vi "Motor_Calibrate.vi"() -> ()   [LabVIEW 2009, in "Motor.lvlib"]
uses:
  Motor.lvlib
  PWM/PWM_Name.ctl
  FPGA.lvlib
  PWM.lvlib
panel:
  in  "stop":bool
  in  "start":bool
  in  "PWM_Channel":T1=1 items=["Invalid"=0, "PWM1"=1, "PWM2"=2, "PWM9"=9, "PWM10"=10]
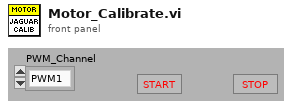
[diagram p1: front panel]
types:
  T1 = typedef "PWM.lvlib/PWM_Name.ctl" = u16
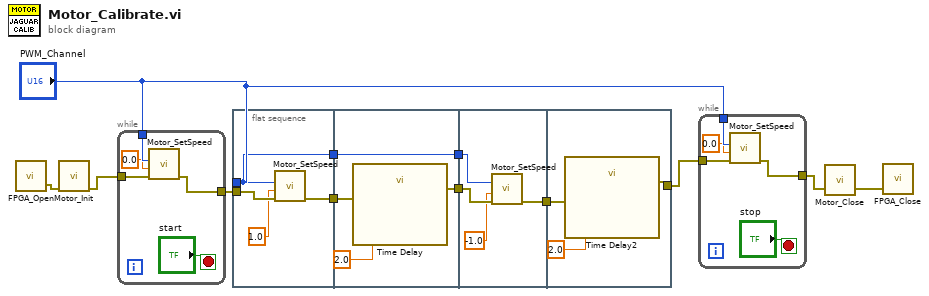
[diagram p0: block diagram]
diagram:
  n1 = call "FPGA_Open.vi"() -> ("error out"=w12:errorcluster)  [unwired: 3 in]
  n2 = call "Motor_Init.vi"("error in"=w12) -> ("error out"=w5:errorcluster)  [unwired: 10 in]
  n3 = while {
    tunnel: w5 -> [w16]
    tunnel: [w15] -> w4
    tunnel: "PWM_Channel" -> [w14]
    stop <- "start" stop-if-true
    n4 = call "Motor_SetSpeed.vi"("error in"=w16, "Speed"=0.0, "PWM_Channel"=w14) -> ("error out"=w15:errorcluster)  [unwired: 8 in]
  }
  n5 = flat-sequence {
    tunnel: w4 -> [w21]
    tunnel: "PWM_Channel" -> [w18]
    tunnel: [w19] -> w10
    tunnel: [w18] -> w7
    tunnel: w10 -> [w25]
    tunnel: [w24] -> w9
    tunnel: [w22] -> w8
    tunnel: w7 -> [w22]
    tunnel: w9 -> [w28]
    tunnel: w8 -> [w29]
    tunnel: [w26] -> w6
    tunnel: [w31] -> w3
    tunnel: w6 -> [w32]
    frame #0 {
      n6 = call "Motor_SetSpeed.vi"("error in"=w21, "Speed"=1.0, "PWM_Channel"=w18) -> ("error out"=w19:errorcluster)  [unwired: 8 in]
    }
    frame #1 {
      n7 = call "Time Delay"("error in (no error)"=w25, "Delay Time (s)"=2.0) -> ("error out"=w24:errorcluster)  [unwired: 9 in]
    }
    frame #2 {
      n8 = call "Motor_SetSpeed.vi"("error in"=w28, "Speed"=-1.0, "PWM_Channel"=w29) -> ("error out"=w26:errorcluster)  [unwired: 8 in]
    }
    frame #3 {
      n9 = call "Time Delay2"("error in (no error)"=w32, "Delay Time (s)"=2.0) -> ("error out"=w31:errorcluster)  [unwired: 9 in]
    }
  }
  n10 = while {
    tunnel: w3 -> [w36]
    tunnel: [w35] -> w2
    tunnel: "PWM_Channel" -> [w34]
    stop <- "stop" stop-if-true
    n11 = call "Motor_SetSpeed.vi"("error in"=w36, "Speed"=0.0, "PWM_Channel"=w34) -> ("error out"=w35:errorcluster)  [unwired: 8 in]
  }
  n12 = call "Motor_Close.vi"("error in"=w2) -> ("error out"=w11:errorcluster)  [unwired: 2 in]
  n13 = call "FPGA_Close.vi"("error in (no error)"=w11) -> ()  [unwired: 2 in, 1 out]
